vi "FABR-Save Data.vi"(1 "State (in)":T6, 5 "Params":T1={"Stimulus"={"Ear"=enum."Left", "Start (kHz)"=0.0, "Stop (kHz)"=16.0, "Step (oct)"=5.0, "Start (dB)"=0, "Stop (dB)"=30, "Step (dB)"=5, "Rep rate (/sec)"=30.0, "Alternate Polarity"=FALSE, "Skip (oct)"=0.0}, "Response"={"Gain"=1.0, "Averages"=0, "Window (ms)"=0.0}, "Hidden"={"AI Samp Rate Hz"=10000.0, "AO Samp Rate Hz"=512.0, "Duration (ms)"=8.5, "Ramp (ms)"=8.5, "Frame size (s)"=0.0}, "Reject"=0.0} {"Response"."Window (ms)" format="%.2f"; "Stimulus"."Start (kHz)" step=5.0; "Stimulus"."Start (dB)" step=5}, 9 "Aborted?":bool, 11 "error in (no error)":errorcluster, 12 "Analysis":T5, 13 "Notes":string) -> (3 "State (out)":T6, 4 "Run #":i16, 10 "Saved?":bool, 15 "error out":errorcluster)   [LabVIEW 2020]
uses:
  CFTS Main Panel SubVIs/CFTS-Experiment State.ctl
  Typedefs/FABR-Analysis State.ctl
  Typedefs/FABR-Parameters.ctl
  Typedefs/FABR-Stimulus.ctl
  Typedefs/FABR-Response.ctl
  Typedefs/FABR-Hidden Params.ctl
  CFTS Main Panel SubVIs/CFTS-Data Type Enum.ctl
  epl-vi-lib/Utility VIs/File IO VIs/Configuration File Wrapper VIs/Config-Read Key (string).vi
panel:
  # "Freq X Level X Time"
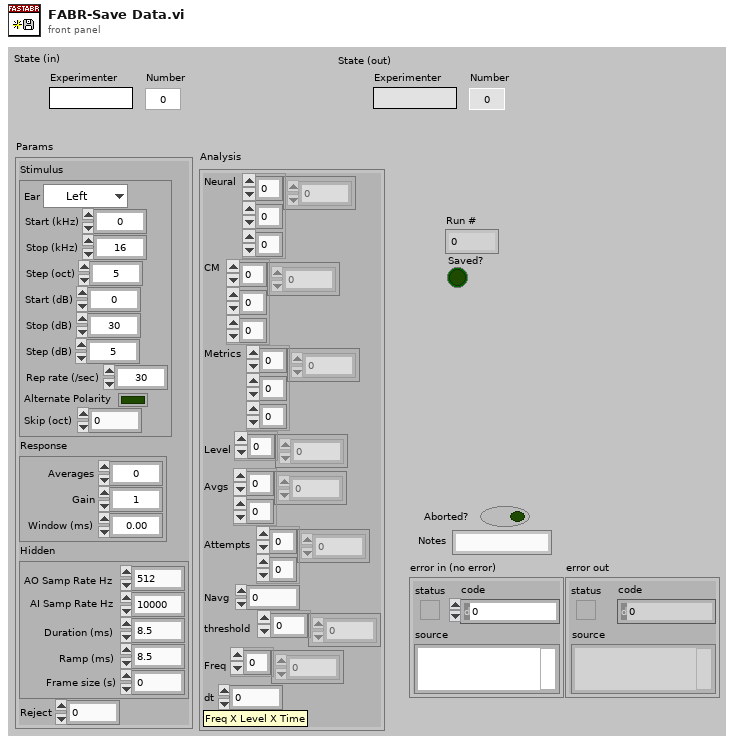
[diagram p1: front panel]
types:
  T1 = typedef "FABR-Parameters.ctl" = cluster{"Stimulus":T2, "Response":T3, "Hidden":T4, "Reject":dbl}
  T2 = typedef "FABR-Stimulus.ctl" = cluster{"Ear":enum16{"Right", "Left"}, "Start (kHz)":dbl, "Stop (kHz)":dbl, "Step (oct)":dbl, "Start (dB)":i32, "Stop (dB)":i32, "Step (dB)":i32, "Rep rate (/sec)":dbl, "Alternate Polarity":bool, "Skip (oct)":dbl}
  T3 = typedef "FABR-Response.ctl" = cluster{"Gain":dbl, "Averages":i32, "Window (ms)":sgl}
  T4 = typedef "FABR-Hidden Params.ctl" = cluster{"AI Samp Rate Hz":dbl, "AO Samp Rate Hz":dbl, "Duration (ms)":dbl, "Ramp (ms)":dbl, "Frame size (s)":dbl}
  T5 = typedef "FABR-Analysis State.ctl" = cluster{"Neural":dbl[][][], "CM":dbl[][][], "Metrics":dbl[][][], "Level":dbl[], "Avgs":i32[][], "Attempts":i32[][], "Navg":i32, "threshold":dbl[], "Freq":dbl[], "dt":dbl}
  T6 = typedef "CFTS-Experiment State.ctl" = cluster{"Experimenter":string, "Number":u32, "Right":string, "Left":string, "Data Folder":path, "State File":path, "Version Info":string, "End Exposure Time":dbl, "Exposure Duration":string, "Run #":cluster{"CAP":i16, "ABR":i16, "DP":i16, "VsEP":i16, "MeasSeq":i16, "SubSeq":i16, "SFOAE":i16}}
  T7 = typedef "CFTS-Data Type Enum.ctl" = enum16{"CAP", "ABR", "DP", "VsEP", "MeasSeq", "SFOAE"}
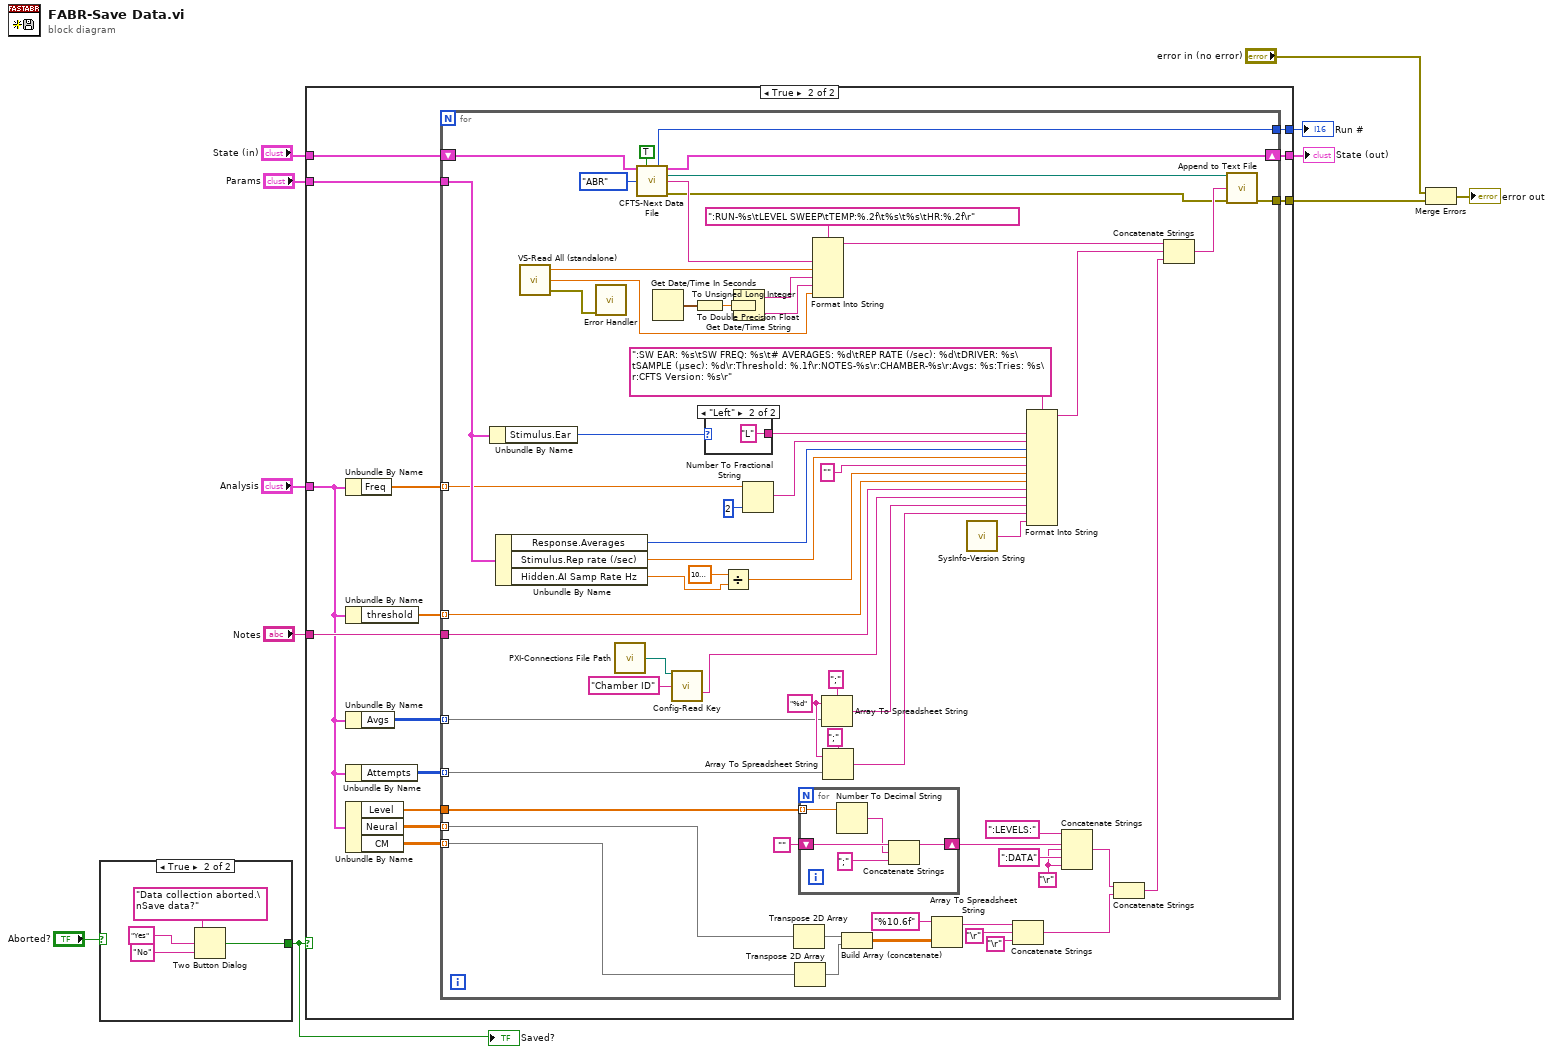
[diagram p0: block diagram]
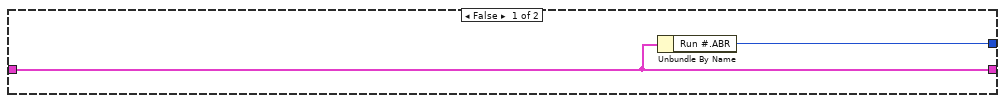
[diagram p2: hidden frame]
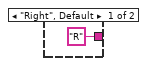
[diagram p3: hidden frame]
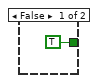
[diagram p4: hidden frame]
diagram:
  n1 = case shown="True" "Aborted?" {
    tunnel: [TRUE ("T button?") w13] -> w7
    frame False {
    }
    frame True {
      n2 = Two Button Dialog(message="Data collection aborted.\nSave data?", 1:"No" ("F button name (\"Cancel\")"), 2:"Yes" ("T button name (\"OK\")")) -> (T button?=w13:bool)
    }
  }
  "Saved?" <- w7
  n3 = case shown="True" w7 {
    tunnel: "State (in)" -> [w18 w32]
    tunnel: [w18 w31] -> w4
    tunnel: "Notes" -> [_ w30]
    tunnel: [w17 w29] -> w9
    tunnel: "Analysis" -> [_ w21]
    tunnel: [_ w28] -> w1
    tunnel: "Params" -> [_ w27]
    frame False {
      n4 = Unbundle By Name(w18) -> ("Run #.ABR"=w17:i16)
    }
    frame True {
      n5 = Unbundle By Name(w21) -> ("Freq"=w26:dbl[])
      n6 = Unbundle By Name(w21) -> ("threshold"=w25:dbl[])
      n7 = Unbundle By Name(w21) -> ("Avgs"=w20:i32[][])
      n8 = Unbundle By Name(w21) -> ("Attempts"=w19:i32[][])
      n9 = Unbundle By Name(w21) -> ("Level"=w24:dbl[], "Neural"=w23:dbl[][][], "CM"=w22:dbl[][][])
      n10 = for {
        tunnel: w30 -> [w76]
        tunnel: [w75] -> w29
        tunnel: [w59] -> w28
        tunnel: w27 -> [w47]
        shift-right: [w96] -> w31
        shift-left: w32 -> [w97]
        tunnel: w26 -> [w39] mode=indexing
        tunnel: w25 -> [w38] mode=indexing
        tunnel: w24 -> [w37]
        tunnel: w23 -> [w36] mode=indexing
        tunnel: w22 -> [w35] mode=indexing
        tunnel: w20 -> [w34] mode=indexing
        tunnel: w19 -> [w33] mode=indexing
        w51 = "%d" ("format string")
        w70 = "\r"
        n11 = Unbundle By Name(w47) -> ("Stimulus.Ear"=w82:enum16{"Right", "Left"})
        n12 = Unbundle By Name(w47) -> ("Response.Averages"=w79:i32, "Stimulus.Rep rate (/sec)"=w78:dbl, "Hidden.AI Samp Rate Hz"=w42:dbl)
        n13 = call "VS-Read All (standalone).vi"() -> ("error out"=w57:errorcluster, "Heart Rate (bpm)"=w56:dbl, "Temperature (C)"=w58:dbl)  [unwired: 3 in]
        n14 = call "Error Handler.vi"("error in (no error)"=w57) -> ()  [unwired: 13 in, 2 out]
        n15 = call "PXI-Connections File Path.vi"() -> ("Path"=w46:path)  [unwired: 1 in]
        n16 = call "CFTS-Next Data File.vi"("Expt State"=w97, "Allow overwrite"=TRUE, "Data Type"=CFTS-Data_Type_Enum."ABR") -> ("Run #"=w75:i16, "Expt State out"=w96:T6, "Datafile path"=w86:path, "run #"=w89:string, "error out"=w84:errorcluster)  [unwired: 8 in]
        n17 = Get Date/Time In Seconds() -> (seconds since 1Jan1904=w93:timestamp)
        n18 = call-poly "Config-Read Key.vi"("configuration file path"=w46, "key"="Chamber ID" ("string")) -> ("value"=w45:string)  [unwired: 10 in, 3 out]
        n19 = To Double Precision Float(number=w93) -> (double precision float=w92:dbl)
        n20 = case shown="\"Left\"" w82 {
          tunnel: ["R" "L"] -> w81
          frame "Right", Default {
          }
          frame "Left" {
          }
        }
        n21 = Divide(x=1000000.0, y=w42) -> (x/y=w41:dbl)
        n22 = To Unsigned Long Integer(number=w92) -> (unsigned 32bit integer=w91:u32)
        n23 = Get Date/Time String(seconds (now)=w91) -> (date string=w94:string, time string=w95:string)  [unwired: 2 in]
        n24 = Number To Fractional String(number=w39, precision (6)=2) -> (F-format string=w80:string)  [unwired: 2 in]
        n25 = Transpose 2D Array(2D array=w36) -> (transposed array=w64:dbl[][])
        n26 = Transpose 2D Array(2D array=w35) -> (transposed array=w63:dbl[][])
        n27 = for {
          shift-right: [w101] -> w71
          shift-left: "" -> [w104]
          tunnel: w37 -> [w100] mode=indexing
          n28 = Number To Decimal String(number=w100) -> (decimal integer string=w103:string)  [unwired: 1 in]
          n29 = Concatenate Strings(w104, w103, ";") -> (w101:string)
        }
        n30 = Format Into String(format string=":RUN-%s\tLEVEL SWEEP\tTEMP:%.2f\t%s\t%s\tHR:%.2f\r", w89, w58, w94, w95, w56) -> (resulting string=w88:string)  [unwired: 2 in, 1 out]
        n31 = Array To Spreadsheet String(delimiter (Tab)=";", array=w34, 3:w51) -> (spreadsheet string=w53:string)
        n32 = Array To Spreadsheet String(delimiter (Tab)=";", array=w33, 3:w51) -> (spreadsheet string=w50:string)
        n33 = Build Array (concatenate)(w64, w63) -> (w62:dbl[][])
        n34 = Array To Spreadsheet String(array=w62, 3:"%10.6f") -> (spreadsheet string=w67:string)  [unwired: 1 in]
        n35 = call "SysInfo-Version String.vi"() -> ("Version String"=w49:string)  [unwired: 1 in]
        n36 = Concatenate Strings(w67, "\r", "\r") -> (w61:string)
        n37 = Format Into String(format string=":SW EAR: %s\tSW FREQ: %s\t# AVERAGES: %d\tREP RATE (/sec): %d\tDRIVER: %s\tSAMPLE (µsec): %d\r:Threshold: %.1f\r:NOTES-%s\r:CHAMBER-%s\r:Avgs: %s:Tries: %s\r:CFTS Version: %s\r", w81, w80, w79, w78, "" ("input 5"), w41, w38, w76, w45, w53, w50, w49) -> (resulting string=w83:string)  [unwired: 2 in, 1 out]
        n38 = Concatenate Strings(":LEVELS:", w71, w70, ":DATA", w70) -> (w69:string)
        n39 = Concatenate Strings(w69, w61) -> (w60:string)
        n40 = Concatenate Strings(w88, w83, w60) -> (w85:string)
        n41 = call "Append to Text File.vi"("file path"=w86, "text"=w85, "error in (no error)"=w84) -> ("error out"=w59:errorcluster)  [unwired: 11 in, 1 out]
      }
    }
  }
  "State (out)" <- w4
  "Run #" <- w9
  n42 = Merge Errors("error in (no error)", w1) -> (→"error out":errorcluster)
